vi "RSxxx Protocol FG.vi"(7 "Action":T1, 8 "error in (no error)":errorcluster, 10 "Serial Config":T2={"Port"="COM1", "Baud Rate"=9600, "Data Bits"=8, "Parity"=enum."None", "Stop Bits"=10, "Flow Control"=0, "XON"=enum."DC1", "XOFF"=enum."DC3", "End Read on Termination Character"=TRUE, "End Write on Termination Character"=TRUE, "Termination Character"=10, "4wireMode"=TRUE, "AssertDTR"=TRUE, "WireMode"=-1} {"WireMode" items=["Unknown"=-1, "RS485/Wire4"=0, "RS485/Wire2-EchoDTR"=1, "RS485/Wire2-CtrlDTR"=2, "RS485/Wire2-Auto"=3, "RS232/DTE"=128, "RS232/DCE"=129, "RS232/Auto"=130]; "Termination Character" format="%.0x"; "Flow Control" items=["None"=0, "XON/XOFF"=1, "RTS/CTS"=2, "DTR/DSR"=4]; "Stop Bits" items=["1.0"=10, "1.5"=15, "2.0"=20]; "Data Bits" min=5 max=8 step=1; "Baud Rate" items=["75"=75, "110"=110, "134"=134, "150"=150, "300"=300, "600"=600, "1200"=1200, "1800"=1800, "2400"=2400, "4800"=4800, "7200"=7200, "9600"=9600, "14400"=14400, "19200"=19200, "28800"=28800, "38400"=38400, "56000"=56000, "57600"=57600, "115200"=115200, "128000"=128000, "230400"=230400, "460800"=460800, "921600"=921600, "1843200"=1843200, "3000000"=3000000]}, 11 "Device Item Ref in":T3 format="%.0x") -> (0 "error out":errorcluster, 2 "Serial Config":T2={"Port"="", "Baud Rate"=0, "Data Bits"=0, "Parity"=enum."None", "Stop Bits"=0, "Flow Control"=0, "XON"=enum."NUL", "XOFF"=enum."NUL", "End Read on Termination Character"=FALSE, "End Write on Termination Character"=FALSE, "Termination Character"=0, "4wireMode"=TRUE, "AssertDTR"=TRUE, "WireMode"=-1} {"WireMode" items=["Unknown"=-1, "RS485/Wire4"=0, "RS485/Wire2-EchoDTR"=1, "RS485/Wire2-CtrlDTR"=2, "RS485/Wire2-Auto"=3, "RS232/DTE"=128, "RS232/DCE"=129, "RS232/Auto"=130]; "Termination Character" format="%.0x"; "Flow Control" items=["None"=0, "XON/XOFF"=1, "RTS/CTS"=2, "DTR/DSR"=4]; "Stop Bits" items=["1.0"=10, "1.5"=15, "2.0"=20]; "Data Bits" min=5 max=8 step=1; "Baud Rate" items=["75"=75, "110"=110, "134"=134, "150"=150, "300"=300, "600"=600, "1200"=1200, "1800"=1800, "2400"=2400, "4800"=4800, "7200"=7200, "9600"=9600, "14400"=14400, "19200"=19200, "28800"=28800, "38400"=38400, "56000"=56000, "57600"=57600, "115200"=115200, "128000"=128000, "230400"=230400, "460800"=460800, "921600"=921600, "1843200"=1843200, "3000000"=3000000]}, 3 "Item Ref out":T3 format="%.0x")   [LabVIEW 2023, in "Instrument Addon Shared.lvlib"]
uses:
  Instrument Addon Shared.lvlib
  <vilib>/NI VeriStand/Custom Device API/Custom Device Item Ref.ctl
  Types/RSXXX Port Settings.ctl
  Types/FG Control.ctl
  Constants.vi
  <vilib>/NI VeriStand/Custom Device API/Get Item Property (U32).vi
  <vilib>/NI VeriStand/Custom Device API/Get Item Property (Boolean).vi
  <vilib>/NI VeriStand/Custom Device API/Get Item Property (String).vi
  <vilib>/NI VeriStand/Custom Device API/Set Item Property (U32).vi
  <vilib>/NI VeriStand/Custom Device API/Set Item Property (Boolean).vi
  <vilib>/NI VeriStand/Custom Device API/Set Item Property (String).vi
  <vilib>/NI VeriStand/Custom Device API/Custom Device API.lvlib
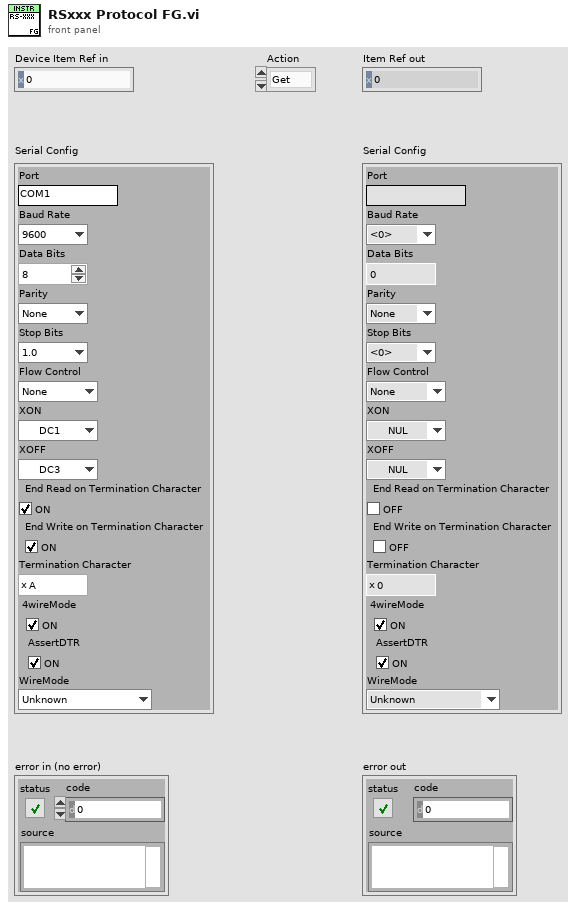
[diagram p1: front panel]
types:
  T1 = typedef "Instrument Addon Shared.lvlib/FG Control.ctl" = enum16{"Get", "Set"}
  T2 = typedef "Instrument Addon Shared.lvlib/RSXXX Port Settings.ctl" = cluster{"Port":string, "Baud Rate":u32, "Data Bits":u16, "Parity":enum16{"None", "Odd", "Even", "Mark", "Space"}, "Stop Bits":u16, "Flow Control":u16, "XON":enum16{"NUL", "SOH", "STX", "ETX", "EOT", "ENQ", "ACK", "BEL", "BS", "HT", "LF", "VT", "FF", "CR", "SO", "SI", "DLE", "DC1", "DC2", "DC3", "DC4", "NAK", "SYN", "ETB", "CAN", "EM", "SUB", "ESC", "FS", "GS", "RS", "US", "SP", "!", "\"", "#", "$", "%", "&", "'", "(", ")", "*", "+", ",", "- (-)", ".", "/", "0", "1", "2", "3", "4", "5", "6", "7", "8", "9", ":", ";", "<", "=", ">", "?", "@", "A", "B", "C", "D", "E", "F", "G", "H", "I", "J", "K", "L", "M", "N", "O", "P", "Q", "R", "S", "T", "U", "V", "W", "X", "Y", "Z", "[", "\\", "]", "^", "_", "`", "a", "b", "c", "d", "e", "f", "g", "h", "i", "j", "k", "l", "m", "n", "o", "p", "q", "r", "s", "t", "u", "v", "w", "x", "y", "z", "{", "|", "}", "~"}, "XOFF":enum16{"NUL", "SOH", "STX", "ETX", "EOT", "ENQ", "ACK", "BEL", "BS", "HT", "LF", "VT", "FF", "CR", "SO", "SI", "DLE", "DC1", "DC2", "DC3", "DC4", "NAK", "SYN", "ETB", "CAN", "EM", "SUB", "ESC", "FS", "GS", "RS", "US", "SP", "!", "\"", "#", "$", "%", "&", "'", "(", ")", "*", "+", ",", "- (-)", ".", "/", "0", "1", "2", "3", "4", "5", "6", "7", "8", "9", ":", ";", "<", "=", ">", "?", "@", "A", "B", "C", "D", "E", "F", "G", "H", "I", "J", "K", "L", "M", "N", "O", "P", "Q", "R", "S", "T", "U", "V", "W", "X", "Y", "Z", "[", "\\", "]", "^", "_", "`", "a", "b", "c", "d", "e", "f", "g", "h", "i", "j", "k", "l", "m", "n", "o", "p", "q", "r", "s", "t", "u", "v", "w", "x", "y", "z", "{", "|", "}", "~"}, "End Read on Termination Character":bool, "End Write on Termination Character":bool, "Termination Character":u8, "4wireMode":bool, "AssertDTR":bool, "WireMode":i16}
  T3 = typedef "Custom Device API.lvlib/Custom Device Item Ref.ctl" = u64
  T4 = enum16{"NUL", "SOH", "STX", "ETX", "EOT", "ENQ", "ACK", "BEL", "BS", "HT", "LF", "VT", "FF", "CR", "SO", "SI", "DLE", "DC1", "DC2", "DC3", "DC4", "NAK", "SYN", "ETB", "CAN", "EM", "SUB", "ESC", "FS", "GS", "RS", "US", "SP", "!", "\"", "#", "$", "%", "&", "'", "(", ")", "*", "+", ",", "- (-)", ".", "/", "0", "1", "2", "3", "4", "5", "6", "7", "8", "9", ":", ";", "<", "=", ">", "?", "@", "A", "B", "C", "D", "E", "F", "G", "H", "I", "J", "K", "L", "M", "N", "O", "P", "Q", "R", "S", "T", "U", "V", "W", "X", "Y", "Z", "[", "\\", "]", "^", "_", "`", "a", "b", "c", "d", "e", "f", "g", "h", "i", "j", "k", "l", "m", "n", "o", "p", "q", "r", "s", "t", "u", "v", "w", "x", "y", "z", "{", "|", "}", "~"}
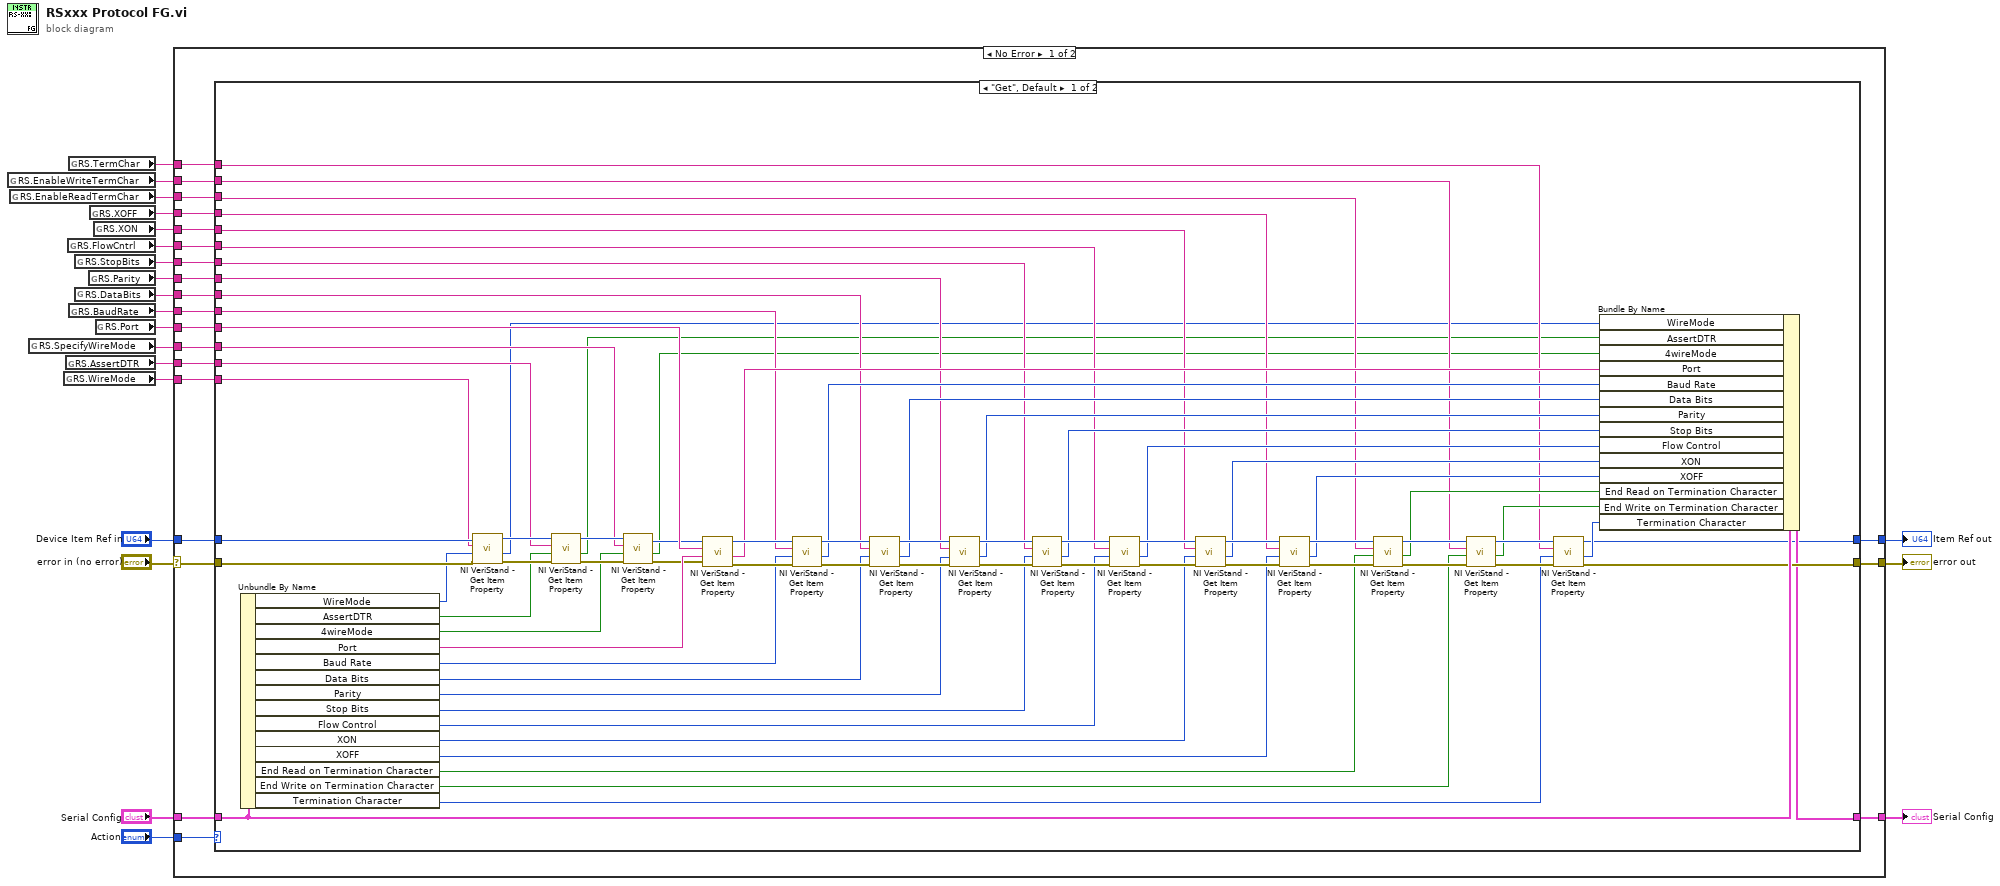
[diagram p0: block diagram]
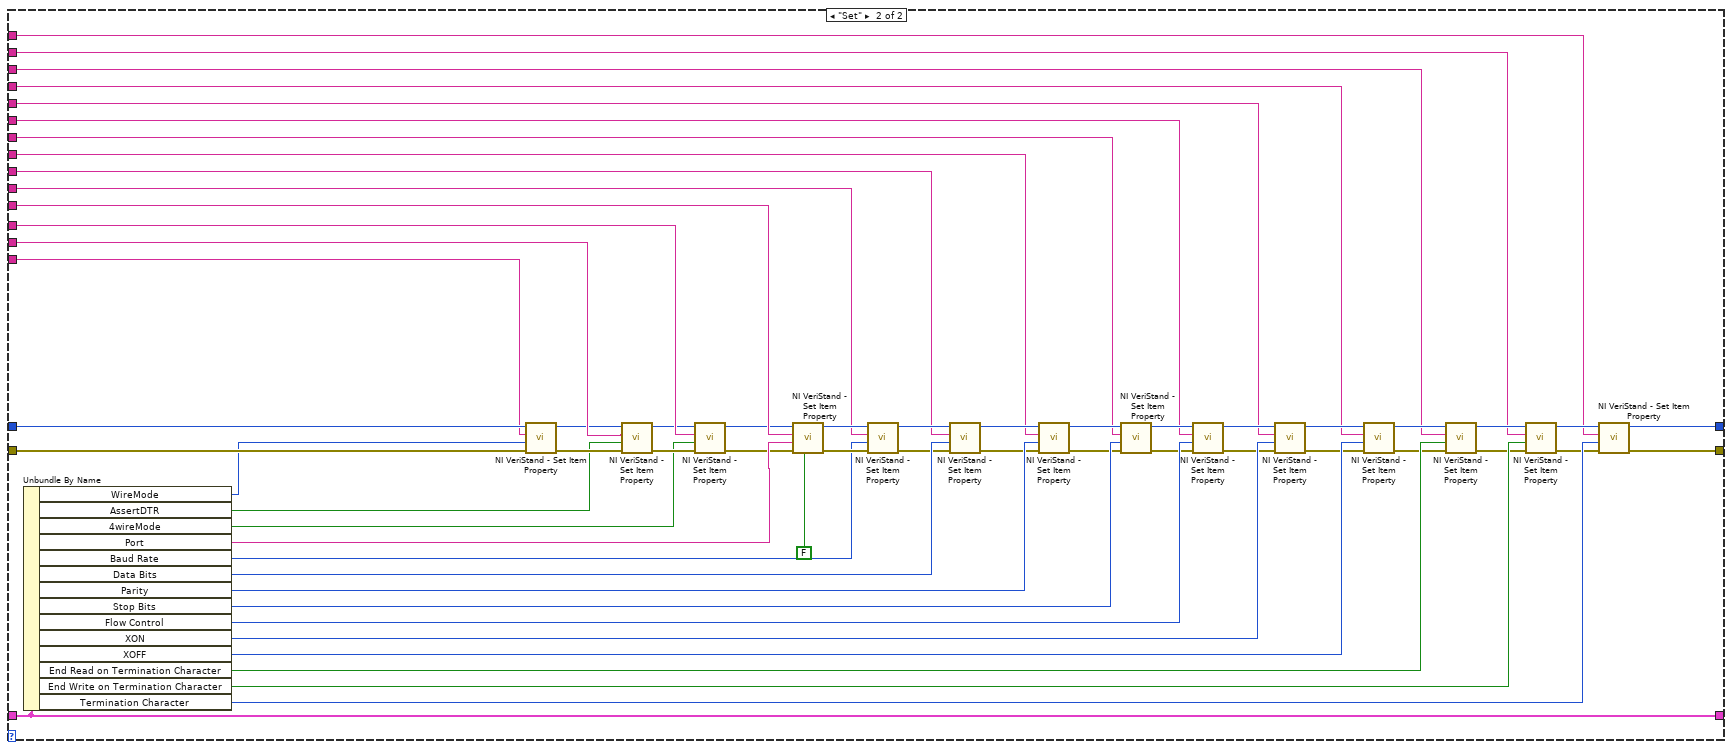
[diagram p2: hidden frame]
diagram:
  n1 = global read "Constants.vi" "RS.EnableWriteTermChar"() -> (w5:string)
  n2 = global read "Constants.vi" "RS.EnableReadTermChar"() -> (w6:string)
  n3 = global read "Constants.vi" "RS.SpecifyWireMode"() -> (w3:string)
  n4 = global read "Constants.vi" "RS.WireMode"() -> (w1:string)
  n5 = global read "Constants.vi" "RS.AssertDTR"() -> (w2:string)
  n6 = global read "Constants.vi" "RS.FlowCntrl"() -> (w9:string)
  n7 = global read "Constants.vi" "RS.TermChar"() -> (w4:string)
  n8 = global read "Constants.vi" "RS.BaudRate"() -> (w13:string)
  n9 = global read "Constants.vi" "RS.StopBits"() -> (w10:string)
  n10 = global read "Constants.vi" "RS.DataBits"() -> (w12:string)
  n11 = global read "Constants.vi" "RS.Parity"() -> (w11:string)
  n12 = global read "Constants.vi" "RS.XOFF"() -> (w7:string)
  n13 = global read "Constants.vi" "RS.XON"() -> (w8:string)
  n14 = global read "Constants.vi" "RS.Port"() -> (w21:string)
  n15 = case shown="No Error" "error in (no error)" {
    selector: "error in (no error)" -> [w37 w179]
    tunnel: w21 -> [w42 _]
    tunnel: [w41 w177] -> w20
    tunnel: "Device Item Ref in" -> [w40 w177]
    tunnel: "Serial Config" -> [w39 w178]
    tunnel: [w38 w179] -> w17
    tunnel: [w36 w178] -> w15
    tunnel: "Action" -> [w35 _]
    tunnel: w13 -> [w34 _]
    tunnel: w12 -> [w33 _]
    tunnel: w11 -> [w32 _]
    tunnel: w10 -> [w31 _]
    tunnel: w9 -> [w30 _]
    tunnel: w8 -> [w29 _]
    tunnel: w7 -> [w28 _]
    tunnel: w6 -> [w27 _]
    tunnel: w5 -> [w26 _]
    tunnel: w4 -> [w25 _]
    tunnel: w3 -> [w24 _]
    tunnel: w2 -> [w23 _]
    tunnel: w1 -> [w22 _]
    frame No Error {
      n16 = case shown="\"Get\", Default" w35 {
        tunnel: w42 -> [w116 w176]
        tunnel: [w70 w132] -> w41
        tunnel: w40 -> [w55 w128]
        tunnel: w39 -> [w84 w175]
        tunnel: [w72 w131] -> w38
        tunnel: w37 -> [w54 w127]
        tunnel: [w71 w175] -> w36
        tunnel: w34 -> [w69 w142]
        tunnel: w33 -> [w68 w141]
        tunnel: w32 -> [w67 w140]
        tunnel: w31 -> [w66 w139]
        tunnel: w30 -> [w65 w138]
        tunnel: w29 -> [w64 w137]
        tunnel: w28 -> [w63 w136]
        tunnel: w27 -> [w62 w135]
        tunnel: w26 -> [w61 w134]
        tunnel: w25 -> [w60 w133]
        tunnel: w24 -> [w51 w124]
        tunnel: w23 -> [w50 w123]
        tunnel: w22 -> [w49 w122]
        frame "Get", Default {
          n17 = Unbundle By Name(w84) -> ("WireMode"=w48:i16, "AssertDTR"=w46:bool, "4wireMode"=w44:bool, "Port"=w115:string, "Baud Rate"=w94:u32, "Data Bits"=w93:u16, "Parity"=w92:enum16{"None", "Odd", "Even", "Mark", "Space"}, "Stop Bits"=w91:u16, "Flow Control"=w90:u16, "XON"=w89:T4, "XOFF"=w88:T4, "End Read on Termination Character"=w87:bool, "End Write on Termination Character"=w86:bool, "Termination Character"=w85:u8)
          n18 = call-poly <vilib>:"NI VeriStand - Get Item Property.vi"("error in (no error)"=w54, "Default Value"=w48, "Property Name"=w49, "Item Ref in"=w55) -> ("error out"=w58:errorcluster, "Value"=w47:u32, "Item Ref out"=w56:T3)  [unwired: 4 in, 1 out]
          n19 = call-poly <vilib>:"NI VeriStand - Get Item Property.vi"("error in (no error)"=w58, "Default Value"=w46, "Property Name"=w50, "Item Ref in"=w56) -> ("error out"=w59:errorcluster, "Value"=w45:bool, "Item Ref out"=w57:T3)  [unwired: 4 in, 1 out]
          n20 = call-poly <vilib>:"NI VeriStand - Get Item Property.vi"("error in (no error)"=w59, "Default Value"=w44, "Property Name"=w51, "Item Ref in"=w57) -> ("error out"=w52:errorcluster, "Value"=w43:bool, "Item Ref out"=w53:T3)  [unwired: 4 in, 1 out]
          n21 = call-poly <vilib>:"NI VeriStand - Get Item Property.vi"("error in (no error)"=w52, "Default Value"=w115, "Property Name"=w116, "Item Ref in"=w53) -> ("error out"=w104:errorcluster, "Value"=w83:string, "Item Ref out"=w114:T3)  [unwired: 4 in, 1 out]
          n22 = call-poly <vilib>:"NI VeriStand - Get Item Property.vi"("error in (no error)"=w104, "Default Value"=w94, "Property Name"=w69, "Item Ref in"=w114) -> ("error out"=w103:errorcluster, "Value"=w82:u32, "Item Ref out"=w113:T3)  [unwired: 4 in, 1 out]
          n23 = call-poly <vilib>:"NI VeriStand - Get Item Property.vi"("error in (no error)"=w103, "Default Value"=w93, "Property Name"=w68, "Item Ref in"=w113) -> ("error out"=w102:errorcluster, "Value"=w81:u32, "Item Ref out"=w112:T3)  [unwired: 4 in, 1 out]
          n24 = call-poly <vilib>:"NI VeriStand - Get Item Property.vi"("error in (no error)"=w102, "Default Value"=w92, "Property Name"=w67, "Item Ref in"=w112) -> ("error out"=w101:errorcluster, "Value"=w80:u32, "Item Ref out"=w111:T3)  [unwired: 4 in, 1 out]
          n25 = call-poly <vilib>:"NI VeriStand - Get Item Property.vi"("error in (no error)"=w101, "Default Value"=w91, "Property Name"=w66, "Item Ref in"=w111) -> ("error out"=w100:errorcluster, "Value"=w79:u32, "Item Ref out"=w110:T3)  [unwired: 4 in, 1 out]
          n26 = call-poly <vilib>:"NI VeriStand - Get Item Property.vi"("error in (no error)"=w100, "Default Value"=w90, "Property Name"=w65, "Item Ref in"=w110) -> ("error out"=w99:errorcluster, "Value"=w78:u32, "Item Ref out"=w109:T3)  [unwired: 4 in, 1 out]
          n27 = call-poly <vilib>:"NI VeriStand - Get Item Property.vi"("error in (no error)"=w99, "Default Value"=w89, "Property Name"=w64, "Item Ref in"=w109) -> ("error out"=w98:errorcluster, "Value"=w77:u32, "Item Ref out"=w108:T3)  [unwired: 4 in, 1 out]
          n28 = call-poly <vilib>:"NI VeriStand - Get Item Property.vi"("error in (no error)"=w98, "Default Value"=w88, "Property Name"=w63, "Item Ref in"=w108) -> ("error out"=w97:errorcluster, "Value"=w76:u32, "Item Ref out"=w107:T3)  [unwired: 4 in, 1 out]
          n29 = call-poly <vilib>:"NI VeriStand - Get Item Property.vi"("error in (no error)"=w97, "Default Value"=w87, "Property Name"=w62, "Item Ref in"=w107) -> ("error out"=w96:errorcluster, "Value"=w75:bool, "Item Ref out"=w106:T3)  [unwired: 4 in, 1 out]
          n30 = call-poly <vilib>:"NI VeriStand - Get Item Property.vi"("error in (no error)"=w96, "Default Value"=w86, "Property Name"=w61, "Item Ref in"=w106) -> ("error out"=w95:errorcluster, "Value"=w74:bool, "Item Ref out"=w105:T3)  [unwired: 4 in, 1 out]
          n31 = call-poly <vilib>:"NI VeriStand - Get Item Property.vi"("error in (no error)"=w95, "Default Value"=w85, "Property Name"=w60, "Item Ref in"=w105) -> ("error out"=w72:errorcluster, "Value"=w73:u32, "Item Ref out"=w70:T3)  [unwired: 4 in, 1 out]
          n32 = Bundle By Name(cluster=w84, "WireMode"=w47, "AssertDTR"=w45, "4wireMode"=w43, "Port"=w83, "Baud Rate"=w82, "Data Bits"=w81, "Parity"=w80, "Stop Bits"=w79, "Flow Control"=w78, "XON"=w77, "XOFF"=w76, "End Read on Termination Character"=w75, "End Write on Termination Character"=w74, "Termination Character"=w73) -> (w71:T2)
        }
        frame "Set" {
          n33 = Unbundle By Name(w175) -> ("WireMode"=w121:i16, "AssertDTR"=w118:bool, "4wireMode"=w117:bool, "Port"=w174:string, "Baud Rate"=w171:u32, "Data Bits"=w169:u16, "Parity"=w168:enum16{"None", "Odd", "Even", "Mark", "Space"}, "Stop Bits"=w167:u16, "Flow Control"=w166:u16, "XON"=w165:T4, "XOFF"=w164:T4, "End Read on Termination Character"=w163:bool, "End Write on Termination Character"=w162:bool, "Termination Character"=w161:u8)
          n34 = call-poly <vilib>:"NI VeriStand - Set Item Property.vi"("error in (no error)"=w127, "Value"=w121, "Property Name"=w122, "Item Ref in"=w128) -> ("error out"=w129:errorcluster, "Item Ref out"=w120:T3)  [unwired: 5 in, 1 out]
          n35 = call-poly <vilib>:"NI VeriStand - Set Item Property.vi"("error in (no error)"=w129, "Value"=w118, "Property Name"=w123, "Item Ref in"=w120) -> ("error out"=w130:errorcluster, "Item Ref out"=w119:T3)  [unwired: 5 in, 1 out]
          n36 = call-poly <vilib>:"NI VeriStand - Set Item Property.vi"("error in (no error)"=w130, "Value"=w117, "Property Name"=w124, "Item Ref in"=w119) -> ("error out"=w125:errorcluster, "Item Ref out"=w126:T3)  [unwired: 5 in, 1 out]
          n37 = call-poly <vilib>:"NI VeriStand - Set Item Property.vi"("Binary String (T)"=FALSE, "error in (no error)"=w125, "Value"=w174, "Property Name"=w176, "Item Ref in"=w126) -> ("error out"=w172:errorcluster, "Item Ref out"=w170:T3)  [unwired: 4 in, 1 out]
          n38 = call-poly <vilib>:"NI VeriStand - Set Item Property.vi"("error in (no error)"=w172, "Value"=w171, "Property Name"=w142, "Item Ref in"=w170) -> ("error out"=w160:errorcluster, "Item Ref out"=w151:T3)  [unwired: 5 in, 1 out]
          n39 = call-poly <vilib>:"NI VeriStand - Set Item Property.vi"("error in (no error)"=w160, "Value"=w169, "Property Name"=w141, "Item Ref in"=w151) -> ("error out"=w159:errorcluster, "Item Ref out"=w150:T3)  [unwired: 5 in, 1 out]
          n40 = call-poly <vilib>:"NI VeriStand - Set Item Property.vi"("error in (no error)"=w159, "Value"=w168, "Property Name"=w140, "Item Ref in"=w150) -> ("error out"=w158:errorcluster, "Item Ref out"=w149:T3)  [unwired: 5 in, 1 out]
          n41 = call-poly <vilib>:"NI VeriStand - Set Item Property.vi"("error in (no error)"=w158, "Value"=w167, "Property Name"=w139, "Item Ref in"=w149) -> ("error out"=w157:errorcluster, "Item Ref out"=w148:T3)  [unwired: 5 in, 1 out]
          n42 = call-poly <vilib>:"NI VeriStand - Set Item Property.vi"("error in (no error)"=w157, "Value"=w166, "Property Name"=w138, "Item Ref in"=w148) -> ("error out"=w156:errorcluster, "Item Ref out"=w147:T3)  [unwired: 5 in, 1 out]
          n43 = call-poly <vilib>:"NI VeriStand - Set Item Property.vi"("error in (no error)"=w156, "Value"=w165, "Property Name"=w137, "Item Ref in"=w147) -> ("error out"=w155:errorcluster, "Item Ref out"=w146:T3)  [unwired: 5 in, 1 out]
          n44 = call-poly <vilib>:"NI VeriStand - Set Item Property.vi"("error in (no error)"=w155, "Value"=w164, "Property Name"=w136, "Item Ref in"=w146) -> ("error out"=w154:errorcluster, "Item Ref out"=w145:T3)  [unwired: 5 in, 1 out]
          n45 = call-poly <vilib>:"NI VeriStand - Set Item Property.vi"("error in (no error)"=w154, "Value"=w163, "Property Name"=w135, "Item Ref in"=w145) -> ("error out"=w153:errorcluster, "Item Ref out"=w144:T3)  [unwired: 5 in, 1 out]
          n46 = call-poly <vilib>:"NI VeriStand - Set Item Property.vi"("error in (no error)"=w153, "Value"=w162, "Property Name"=w134, "Item Ref in"=w144) -> ("error out"=w152:errorcluster, "Item Ref out"=w143:T3)  [unwired: 5 in, 1 out]
          n47 = call-poly <vilib>:"NI VeriStand - Set Item Property.vi"("error in (no error)"=w152, "Value"=w161, "Property Name"=w133, "Item Ref in"=w143) -> ("error out"=w131:errorcluster, "Item Ref out"=w132:T3)  [unwired: 5 in, 1 out]
        }
      }
    }
    frame Error {
    }
  }
  "Item Ref out" <- w20
  "error out" <- w17
  "Serial Config" <- w15
